vi "lectura de potenciometro.vi"() -> ()   [LabVIEW 2016]
uses:
  <vilib>/LabVIEW Interface for Arduino/Type Defs/Board Type.ctl
  <vilib>/LabVIEW Interface for Arduino/Type Defs/Connection Type.ctl
  <vilib>/LabVIEW Interface for Arduino/LabVIEW Interface for Arduino.lvlib
panel:
  in  "Stop":bool
  out "Voltaje":dbl(knob) scale=0.0..5.0
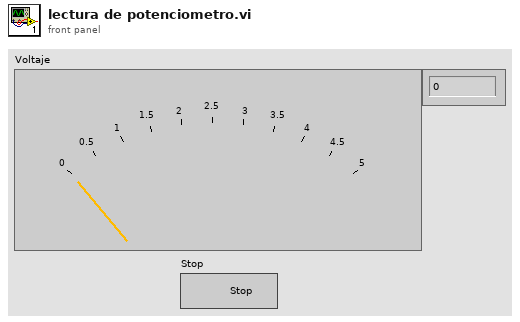
[diagram p1: front panel]
types:
  T1 = typedef "LabVIEW Interface for Arduino.lvlib/Connection Type.ctl" = enum8{"USB / Serial", "XBEE", "BlueSmirf (Bluetooth)"}
  T2 = typedef "LabVIEW Interface for Arduino.lvlib/Board Type.ctl" = enum16{"Uno", "Dimuelanove w/Atmega 328", "Mega 2560"}
  T3 = typedef "LabVIEW Interface for Arduino.lvlib/Arduino Resource.ctl" = cluster{"VISA resource":refnum<visa-resource-name>, "Board Type":T2, "Connection Type":enum8{"USB / Serial"}, "Bytes Per Packet (15)":u8}
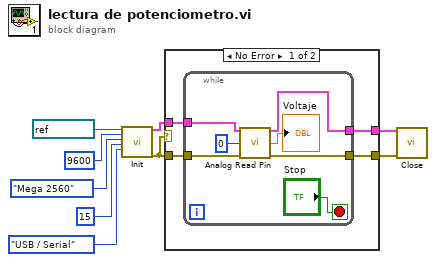
[diagram p0: block diagram]
diagram:
  n1 = call <vilib>:"Init.vi"("VISA resource"=refnum<visa-resource-name> "COM6", "Baud Rate (115200)"=u32 9600, "Board Type (Uno)"=Board_Type."Mega 2560", "Bytes Per Packet (15)"=u32 15, "Connection Type (USB/Serial)"=Connection_Type."USB / Serial") -> ("Arduino Resource"=w4:T3, "error out"=w3:errorcluster)  [unwired: 13 in]
  n2 = case shown="No Error" w3 {
    tunnel: w4 -> [w13 w22]
    tunnel: w3 -> [w12 w21]
    tunnel: [w10 w21] -> w2
    tunnel: [w11 w22] -> w1
    frame No Error {
      n3 = while {
        tunnel: w13 -> [w19]
        tunnel: [w16] -> w11
        tunnel: [w15] -> w10
        tunnel: w12 -> [w14]
        stop <- "Stop" stop-if-true
        n4 = call <vilib>:"Analog Read Pin.vi"("Arduino Resource"=w19, "Analog Input Pin (0)"=u8 0, "error in"=w14) -> ("Arduino Resource"=w16:T3, "Voltage"=→"Voltaje":dbl, "error out"=w15:errorcluster)  [unwired: 10 in]
      }
    }
    frame Error {
    }
  }
  n5 = call <vilib>:"Close.vi"("Arduino Resource"=w1, "error in"=w2) -> ()  [unwired: 13 in, 1 out]
